vi "CSM - List Rules in Broadcast Registry.vi"(8 "error in (no error)":errorcluster) -> (0 "error out":errorcluster, 3 "Entries":T1(array[cluster]))   [LabVIEW 2020, in "Communicable State Machine.lvlib"]
uses:
  Communicable State Machine.lvlib
  Operation-BroadcastRegistry.ctl
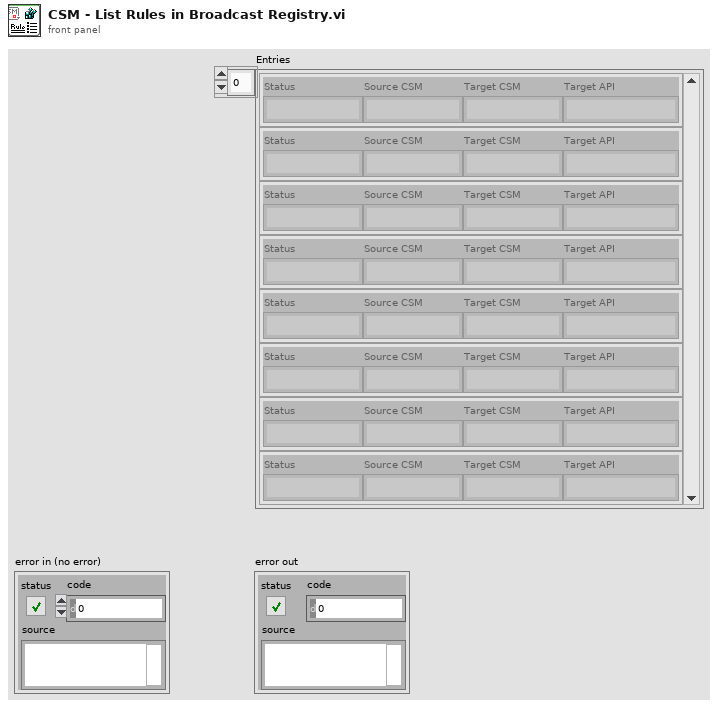
[diagram p1: front panel]
types:
  T1 = cluster{"Status":string, "Source CSM":string, "Target CSM":string, "Target API":string}[]
  T2 = typedef "Communicable State Machine.lvlib/Operation-BroadcastRegistry.ctl" = enum16{"Delete Source Module", "Delete Target Module", "Remove Module", "Register", "Unregister", "Check", "List Status", "List Entries"}
  T3 = cluster{"Status":string, "Source CSM":string, "Target CSM":string, "Target API":string}
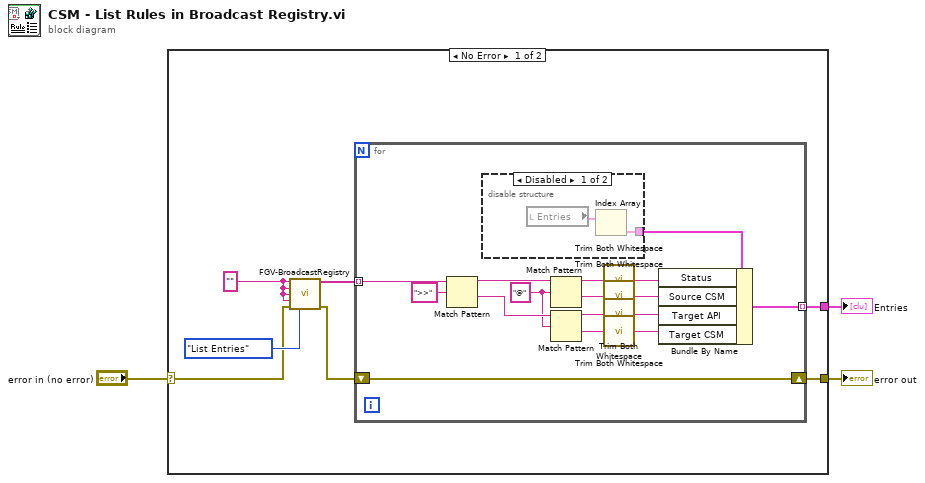
[diagram p0: block diagram]
diagram:
  n1 = case shown="No Error" "error in (no error)" {
    selector: "error in (no error)" -> [w8 w29]
    tunnel: [w10 w29] -> w3
    tunnel: [w4 _] -> w1
    frame No Error {
      w6 = "" ("Source")
      n2 = call "FGV-BroadcastRegistry.vi"("Source"=w6, "Target"=w6, "Status"=w6, "API"=w6, "Error in"=w8, "Operation"=Operation-BroadcastRegistry."List Entries") -> ("response message"=w5:string[], "Error out"=w7:errorcluster)  [unwired: 8 in]
      n3 = for {
        shift-right: [w26] -> w10
        shift-left: w7 -> [w26]
        tunnel: w5 -> [w25] mode=indexing
        tunnel: [w19] -> w4 mode=indexing
        w21 = "@" ("regular expression")
        n4 = Match Pattern(string=w25, regular expression=">>") -> (before substring=w23:string, after substring=w22:string)  [unwired: 1 in, 2 out]
        n5 = disable-structure shown="Disabled" {
          disable-tunnel: [w27 _] -> w20
          frame Disabled {
            n6 = local read "Entries"() -> (w28:T1)
            n7 = Index Array(array=w28) -> (element=w27:T3)  [unwired: 1 in]
          }
          frame Enabled {
          }
        }
        n8 = Match Pattern(string=w23, regular expression=w21) -> (before substring=w18:string, after substring=w17:string)  [unwired: 1 in, 2 out]
        n9 = Match Pattern(string=w22, regular expression=w21) -> (before substring=w16:string, after substring=w15:string)  [unwired: 1 in, 2 out]
        n10 = call "Trim Both Whitespace.vi"("string"=w18) -> ("trimmed string"=w11:string)  [unwired: 1 in]
        n11 = call "Trim Both Whitespace.vi"("string"=w17) -> ("trimmed string"=w12:string)  [unwired: 1 in]
        n12 = call "Trim Both Whitespace.vi"("string"=w16) -> ("trimmed string"=w13:string)  [unwired: 1 in]
        n13 = call "Trim Both Whitespace.vi"("string"=w15) -> ("trimmed string"=w14:string)  [unwired: 1 in]
        n14 = Bundle By Name(cluster=w20, "Status"=w11, "Source CSM"=w12, "Target API"=w13, "Target CSM"=w14) -> (w19:T3)
      }
    }
    frame Error {
    }
  }
  "Entries" <- w1
  "error out" <- w3
